vi "Log (Parts).vi"(7 "log level":T1=enum."Critical", 9 "data (null)":variant, 10 "message":string, 11 "logger in":refnum<class "Logger.lvclass">) -> (3 "logger out":refnum<class "Logger.lvclass">)   [LabVIEW 2018, in "GLog.lvlib" / "Logger.lvclass"]
uses:
  Logger.lvclass
  Log Levels.ctl
  Internal Log Levels.ctl
  GLog.lvlib
panel:
  # "Connector Pane"
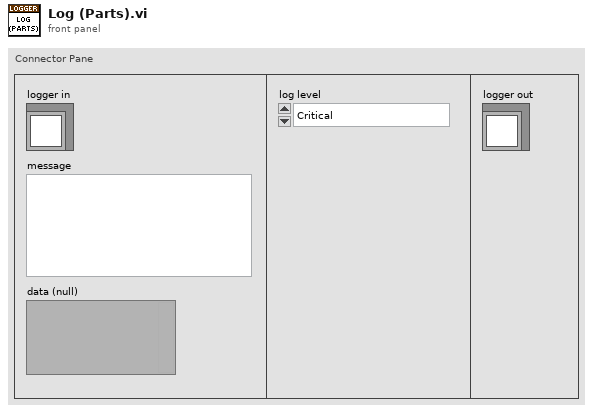
[diagram p1: front panel]
types:
  T1 = typedef "GLog.lvlib/Log Levels.ctl" = enum16{"Trace", "Debug", "Info", "Warning", "Error", "Critical"}
  T2 = typedef "GLog.lvlib/Internal Log Levels.ctl" = enum16{"Trace", "Debug", "Info", "Warning", "Error", "Critical", "Internal"}
  T3 = typedef "GLog.lvlib/Log Record.ctl" = cluster{"level":T2, "timestamp":timestamp, "call chain":string[], "message":string, "data":variant}
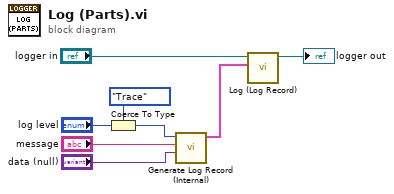
[diagram p0: block diagram]
diagram:
  n1 = Coerce To Type(0:"log level", 1:Internal_Log_Levels."Trace" ("internal log level")) -> (2:w3:T2)
  n2 = call "Generate Log Record (Internal).vi"("data (null)"="data (null)", "message (\"\")"="message", "level (Internal)"=w3) -> ("log record"=w1:T3)  [unwired: 8 in]
  n3 = call "Log (Log Record).vi"("log record"=w1, "Logger in"="logger in") -> ("Logger out"=→"logger out":refnum<class "Logger.lvclass">)  [unwired: 9 in]
